vi "DAQ.Init.vi"(8 "error in (no error)":errorcluster, 11 "DAQmx in":refnum<class "DAQmx.lvclass">) -> (0 "error out":errorcluster, 3 "DAQmx out":refnum<class "DAQmx.lvclass">)   [LabVIEW 2016, in "DAQmx.lvclass"]
uses:
  DAQmx.lvclass
  DAQmx.lvclass/DAQmx.ctl
  <vilib>/DAQmx/write.llb/DAQmx Write (Analog 1D Wfm NChan NSamp).vi
  <vilib>/DAQmx/create/channels.llb/DAQmx Create Channel (AI-Voltage-Basic).vi
  <vilib>/DAQmx/configure/timing.llb/DAQmx Timing (Sample Clock).vi
  <vilib>/DAQmx/create/channels.llb/DAQmx Create Channel (AO-Voltage-Basic).vi
  <vilib>/DAQmx/miscellaneous.llb/DAQmx Fill In Error Info.vi
  <resource>/objmgr/daqmx.rc
  <vilib>/measure/NI_MABase.lvlib
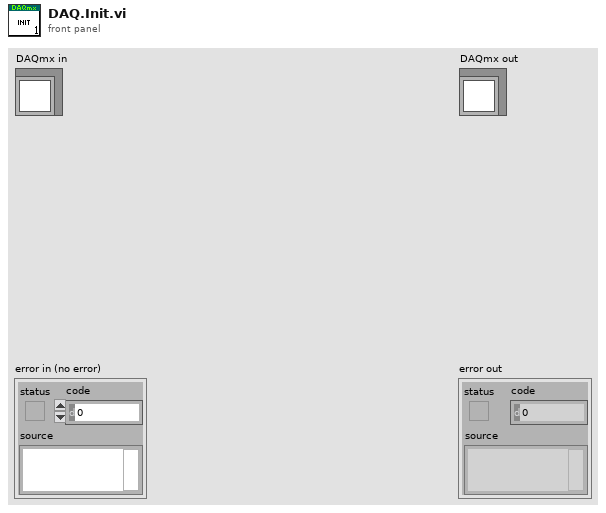
[diagram p1: front panel]
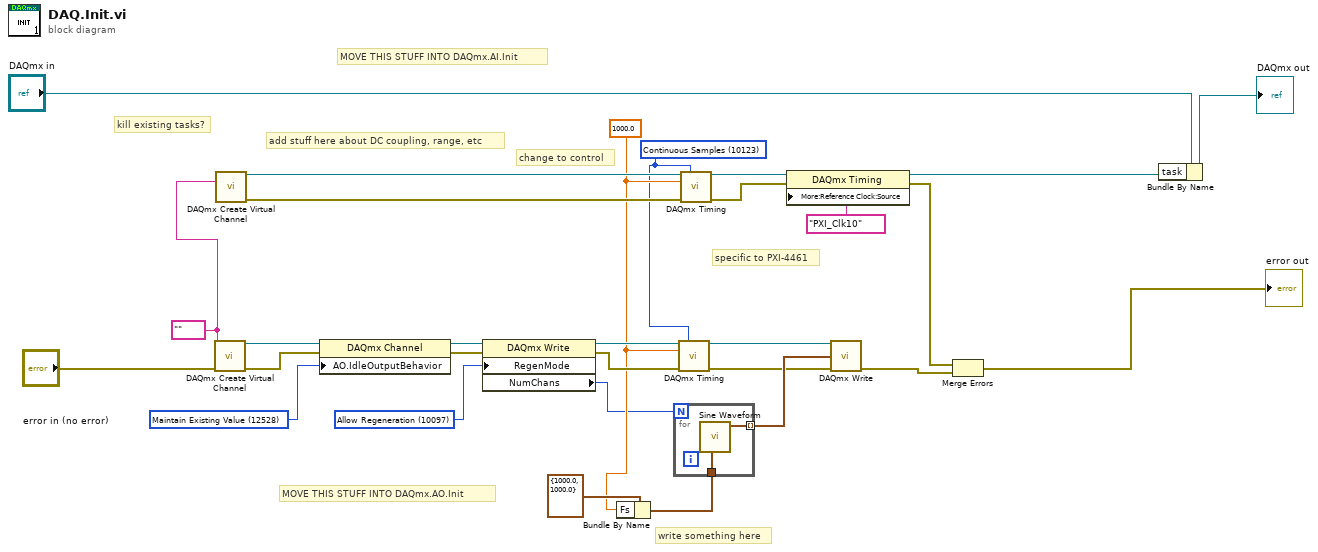
[diagram p0: block diagram]
diagram:
  w1 = tag "" ("physical channels")
  w3 = 10123 items=["Finite Samples"=10178, "Continuous Samples"=10123, "Hardware Timed Single Point"=12522] ("sample mode")
  w5 = 10097 items=["Allow Regeneration"=10097, "Do Not Allow Regeneration"=10158] ("RegenMode")
  w6 = 12528 items=["Zero Volts"=12526, "High-Impedance"=12527, "Maintain Existing Value"=12528] ("AO.IdleOutputBehavior")
  w7 = 1000.0 ("rate")
  # "MOVE THIS STUFF INTO DAQmx.AO.Init"
  # "MOVE THIS STUFF INTO DAQmx.AI.Init"
  # "kill existing tasks?"
  # "write something here"
  # "add stuff here about DC coupling, range, etc"
  # "specific to PXI-4461"
  # "change to control"
  n1 = call-poly <vilib>:"DAQmx Create Virtual Channel.vi"("physical channels"=w1, "error in"="error in (no error)") -> ("task out"=w23:refnum<k21>, "error out"=w22:errorcluster)  [unwired: 12 in]
  n2 = call-poly <vilib>:"DAQmx Create Virtual Channel.vi"("physical channels"=w1) -> ("task out"=w28:refnum<k21>, "error out"=w27:errorcluster)  [unwired: 13 in]
  n3 = property class="DAQmx Channel"(reference=w23, error in=w22, "AO.IdleOutputBehavior"=w6) -> (reference out=w24:refnum<k21>, error out=w25:errorcluster)
  n4 = property class="DAQmx Write"(reference=w24, error in=w25, "RegenMode"=w5) -> (reference out=w21:refnum<k21>, error out=w20:errorcluster, "NumChans"=w4:u32)
  n5 = Bundle By Name(cluster=cluster{"Fs":dbl, "#s":dbl} {"Fs"=1000.0, "#s"=1000.0} ("sampling info"), "Fs"=w7) -> (w17:cluster{"Fs":dbl, "#s":dbl})
  n6 = for {
    N: w4 -> [_]
    tunnel: w17 -> [w31]
    tunnel: [w30] -> w16 mode=indexing
    n7 = call <vilib>:"Sine Waveform.vi"("sampling info"=w31) -> ("signal out"=w30:waveform(dbl))  [unwired: 9 in, 1 out]
  }
  n8 = call-poly <vilib>:"DAQmx Timing.vi"("task/channels in"=w21, "sample mode"=w3, "rate"=w7, "error in"=w20) -> ("task out"=w19:refnum<k21>, "error out"=w15:errorcluster)  [unwired: 10 in]
  n9 = call-poly <vilib>:"DAQmx Timing.vi"("task/channels in"=w28, "sample mode"=w3, "rate"=w7, "error in"=w27) -> ("task out"=w29:refnum<k21>, "error out"=w14:errorcluster)  [unwired: 10 in]
  n10 = property class="DAQmx Timing"(reference=w29, error in=w14, "More:Reference Clock:Source"=tag "PXI_Clk10" ("RefClk.Src")) -> (reference out=w10:refnum<k21>, error out=w13:errorcluster)
  n11 = call-poly <vilib>:"DAQmx Write.vi"("task/channels in"=w19, "data"=w16, "error in"=w15) -> ("error out"=w12:errorcluster)  [unwired: 10 in, 2 out]
  n12 = Merge Errors(w13, w12) -> (→"error out":errorcluster)
  n13 = Bundle By Name(cluster="DAQmx in", "task"=w10) -> (→"DAQmx out":refnum<class "DAQmx.lvclass">)
